vi "c_ctre_phoenix6_platform_set_logger_path.vi"(0 "String 2":string) -> (20 "Numeric":i32, 21 "String":string)   [LabVIEW 2023]
uses:
  <vilib>/Rock Robotics/WPI/ThirdParty/Phoenix-LabVIEW/Controls/DriverLib.ctl
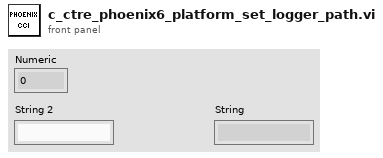
[diagram p1: front panel]
types:
  T1 = typedef "DriverLib.ctl" = path
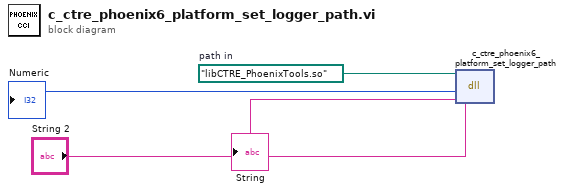
[diagram p0: block diagram]
diagram:
  w4 = T1 path "libCTRE_PhoenixTools.so"  # path in
  n1 = dll-call lib="?" fn="c_ctre_phoenix6_platform_set_logger_path"(path in=w4, "String 2") -> (→"Numeric":i32, →"String":string)  [unwired: 2 in, 2 out]
